vi "WPI_CompressorGetEnableState.vi"(8 "error in (no error)":errorcluster, 11 "CompressorDevRef":T1) -> (0 "error out":errorcluster, 1 "Compressor Running":bool, 2 "Enabled":bool, 3 "CompressorDevRef":T1)   [LabVIEW 2017]
doc: "Returns the enabled state of the compressor and the on/off state of COMPRESSOR OUT on the Pneumatic Control Module.\n\nThis software is licensed. Open the labview\\readme\\WPI Robotics Library Open Source License.txt file for more information."
uses:
  <vilib>/Rock Robotics/WPI/Compressor/WPI_CompressorDevRef.ctl
  <vilib>/Rock Robotics/WPI/CAN/PCM/WPI_CAN_PCMGlobalOps.ctl
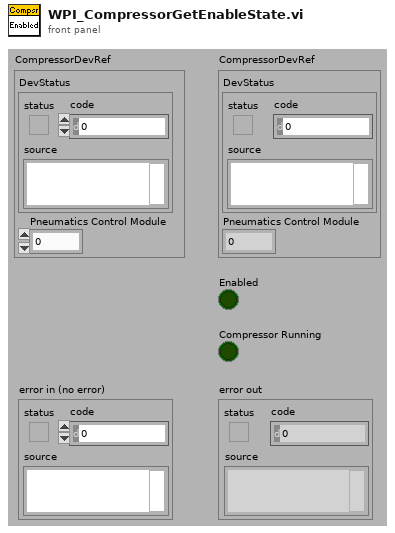
[diagram p1: front panel]
types:
  T1 = typedef "WPI_CompressorDevRef.ctl" = cluster{"DevStatus":errorcluster, "Pneumatics Control Module":u8}
  T2 = typedef "WPI_CAN_PCMGlobalOps.ctl" = enum16{"Read For Send", "Write After Receive", "Set Solenoids", "Set Closed Loop", "Clear Sticky Faults", "Get All", "Write Error", "Write After Receive Blacklist", "Set Control Frame Rate"}
  T3 = cluster{"Solenoid Status":bool[], "Battery Voltage":dbl, "Solenoid Voltage":dbl, "Compressor Current":dbl, "CompressorEnabled":bool, "StickySolenoidFault":bool, "StickyCompressorFault":bool, "SolenoidFault":bool, "CompressorFault":bool, "HardwareFault":bool, "ClosedLoopStatus":bool, "PressureStatus":bool, "Module Enabled":bool, "ClosedLoopSuggestedOutput":bool, "CAN Error":errorcluster, "Sticky Solenoid Faults":bool[]}
  T4 = cluster{"Solenoids":bool[], "Closed Loop Enable":bool, "Clear Sticky Faults":bool, "Control Frame Rate Ms":i32}
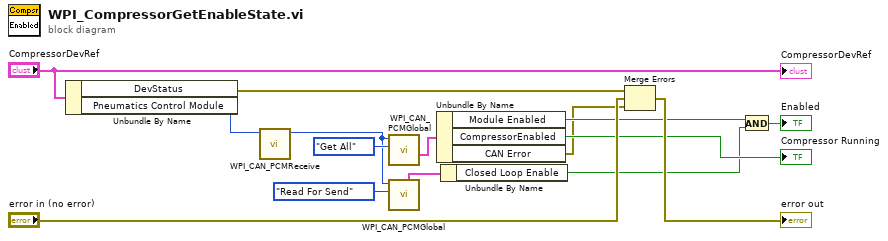
[diagram p0: block diagram]
diagram:
  n1 = Unbundle By Name("CompressorDevRef") -> ("DevStatus"=w15:errorcluster, "Pneumatics Control Module"=w2:u8)
  n2 = call <vilib>:"WPI_CAN_PCMReceive.vi"("Pneumatics Control Module (0)"=w2) -> ("Pneumatics Control Module Out"=w3:u8)  [unwired: 10 in]
  n3 = call <vilib>:"WPI_CAN_PCMGlobal.vi"("Operation"=WPI_CAN_PCMGlobalOps."Get All", "Pneumatics Control Module (0)"=w3) -> ("Get All"=w11:T3)  [unwired: 7 in, 2 out]
  n4 = call <vilib>:"WPI_CAN_PCMGlobal.vi"("Operation"=WPI_CAN_PCMGlobalOps."Read For Send", "Pneumatics Control Module (0)"=w3) -> ("Read For Send"=w6:T4)  [unwired: 7 in, 2 out]
  n5 = Unbundle By Name(w11) -> ("Module Enabled"=w8:bool, "CompressorEnabled"=→"Compressor Running":bool, "CAN Error"=w4:errorcluster)
  n6 = Unbundle By Name(w6) -> ("Closed Loop Enable"=w5:bool)
  n7 = Merge Errors(w15, "error in (no error)", w4) -> (→"error out":errorcluster)
  n8 = And(x=w8, y=w5) -> (x .and. y?=→"Enabled":bool)
  "CompressorDevRef" <- "CompressorDevRef"
